vi "Constructor by Table Config.vi"(8 "error in (no error)":errorcluster, 10 "Table Configuration":refnum<class "Table Configuration Interface.lvclass">, 11 "Form from Table Configuration in":refnum<class "Form from Table Configuration.lvclass">) -> (0 "error out":errorcluster, 3 "Form from Table Configuration out":refnum<class "Form from Table Configuration.lvclass">)   [LabVIEW 2020, in "Panel Form Controller.lvlib" / "Form from Table Configuration.lvclass"]
uses:
  Form from Table Configuration.lvclass
  Database OOP/Table Libraries/Table Configuration Interface/Table Configuration Interface.lvclass
  Form from Table Configuration.lvclass/Form from Table Configuration.ctl
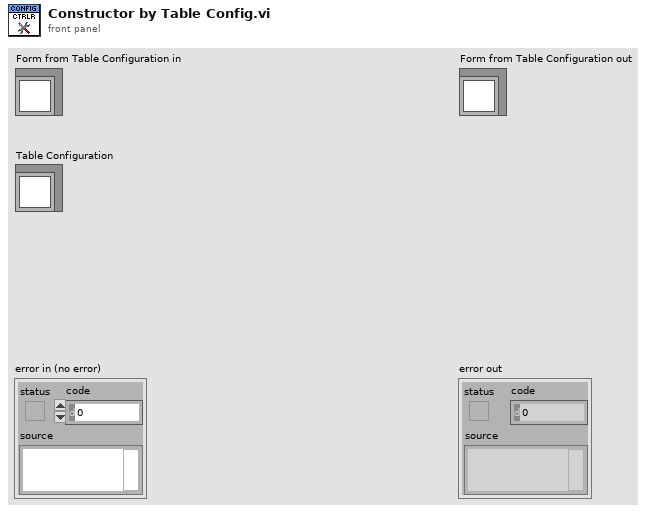
[diagram p1: front panel]
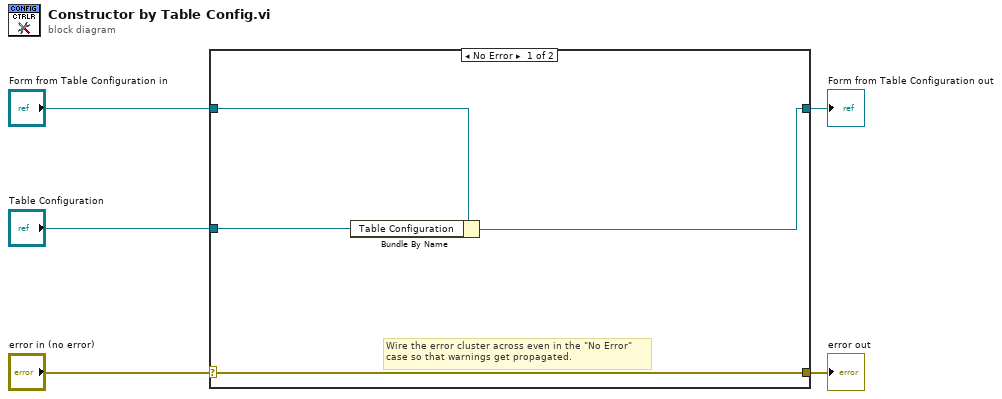
[diagram p0: block diagram]
diagram:
  n1 = case shown="No Error" "error in (no error)" {
    selector: "error in (no error)" -> [w9 w11]
    tunnel: [w9 w11] -> w4
    tunnel: [w6 w10] -> w2
    tunnel: "Form from Table Configuration in" -> [w8 w10]
    tunnel: "Table Configuration" -> [w7 _]
    frame No Error {
      # "Wire the error cluster across even in the \"No Error\"\ncase so that warnings get propagated."
      n2 = Bundle By Name(cluster=w8, "Table Configuration"=w7) -> (w6:refnum<class "Form from Table Configuration.lvclass">)
    }
    frame Error {
    }
  }
  "error out" <- w4
  "Form from Table Configuration out" <- w2
